vi "Array Result Comparison.vi"(7 "Comparison Method":T1, 9 "Values Array to Compare":dbl[][](array[numeric]), 10 "Limit Values Array":dbl[][](array[numeric])) -> (0 "Error Out":errorcluster, 2 "Result":bool caption="Result [True = Pass]")   [LabVIEW 2014]
uses:
  CustomControls/Array_Comparison_Types.ctl
panel:
  in  "Error In":errorcluster
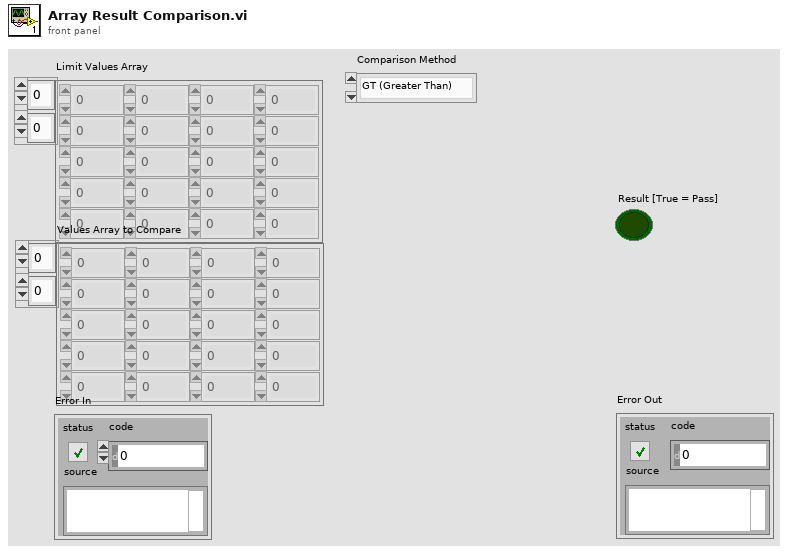
[diagram p1: front panel]
types:
  T1 = typedef "Array_Comparison_Types.ctl" = enum16{"GT (Greater Than)", "LT (Less Than)"}
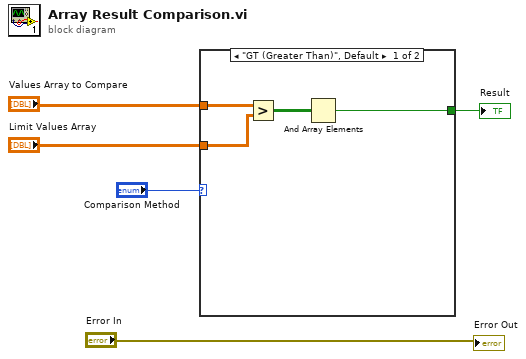
[diagram p0: block diagram]
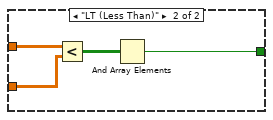
[diagram p2: hidden frame]
diagram:
  n1 = case shown="\"GT (Greater Than)\", Default" "Comparison Method" {
    tunnel: "Values Array to Compare" -> [w9 w13]
    tunnel: "Limit Values Array" -> [w8 w12]
    tunnel: [w6 w10] -> w2
    frame "GT (Greater Than)", Default {
      n2 = Greater?(x=w9, y=w8) -> (0:w7:bool[][])
      n3 = And Array Elements(Boolean array=w7) -> (logical AND=w6:bool)
    }
    frame "LT (Less Than)" {
      n4 = Less?(x=w13, y=w12) -> (x < y?=w11:bool[][])
      n5 = And Array Elements(Boolean array=w11) -> (logical AND=w10:bool)
    }
  }
  "Result" <- w2
  "Error Out" <- "Error In"
